vi "Load Becker-Hickl File Setup.vi"(8 "Error In":errorcluster, 9 "Setup Length":i16, 10 "Setup Offset":i32, 11 "File Path Control":path) -> (0 "Error Out":errorcluster, 1 "TAC Parameters":T3 {"Frequency (Hz)" format="%#.6g"; "TAC Range (s)" format="%.6g"; "TAC Bin (s)" format="%#.6g"}, 2 "Image Parameters":T2, 3 "File Path out":path, 4 "Image Sizes":T1)   [LabVIEW 2021, in "Becker-Hickl Files.lvlib"]
uses:
  Becker-Hickl Files.lvlib
  Becker-Hickl TAC Parameters.ctl
  Becker-Hickl Image Parameters.ctl
  Becker-Hickl FLIM Image Sizes.ctl
panel:
  out "Setup Binary Data String":string
  out "Setup Data String":string
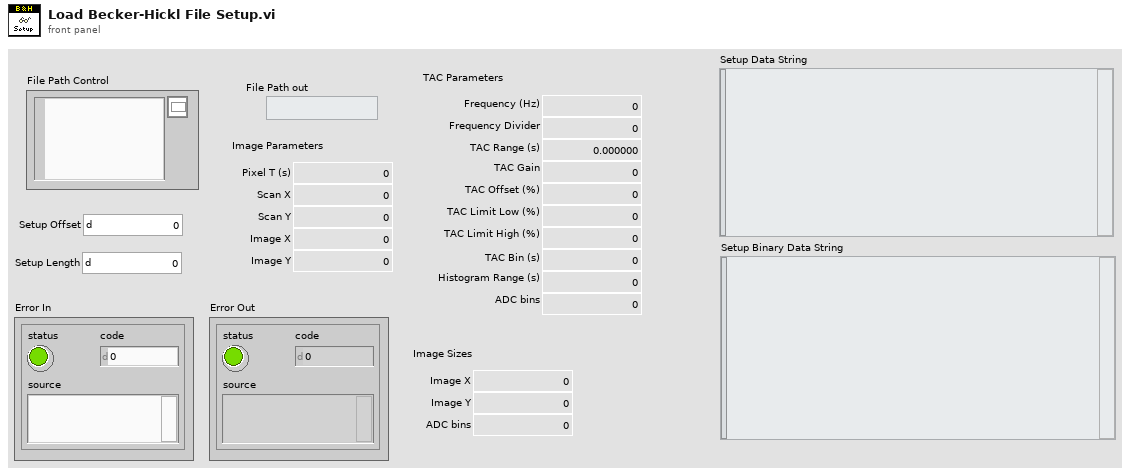
[diagram p1: front panel]
types:
  T1 = typedef "Becker-Hickl Files.lvlib/Becker-Hickl FLIM Image Sizes.ctl" = cluster{"Image X":i32, "Image Y":i32, "ADC bins":i32}
  T2 = typedef "Becker-Hickl Files.lvlib/Becker-Hickl Image Parameters.ctl" = cluster{"Pixel T (s)":dbl, "Scan X":i32, "Scan Y":i32, "Image X":i32, "Image Y":i32}
  T3 = typedef "Becker-Hickl Files.lvlib/Becker-Hickl TAC Parameters.ctl" = cluster{"Frequency (Hz)":dbl, "Frequency Divider":i32, "TAC Range (s)":dbl, "TAC Gain":i32, "TAC Offset (%)":dbl, "TAC Limit Low (%)":dbl, "TAC Limit High (%)":dbl, "TAC Bin (s)":dbl, "ADC bins":i32, "Histogram Range (s)":dbl}
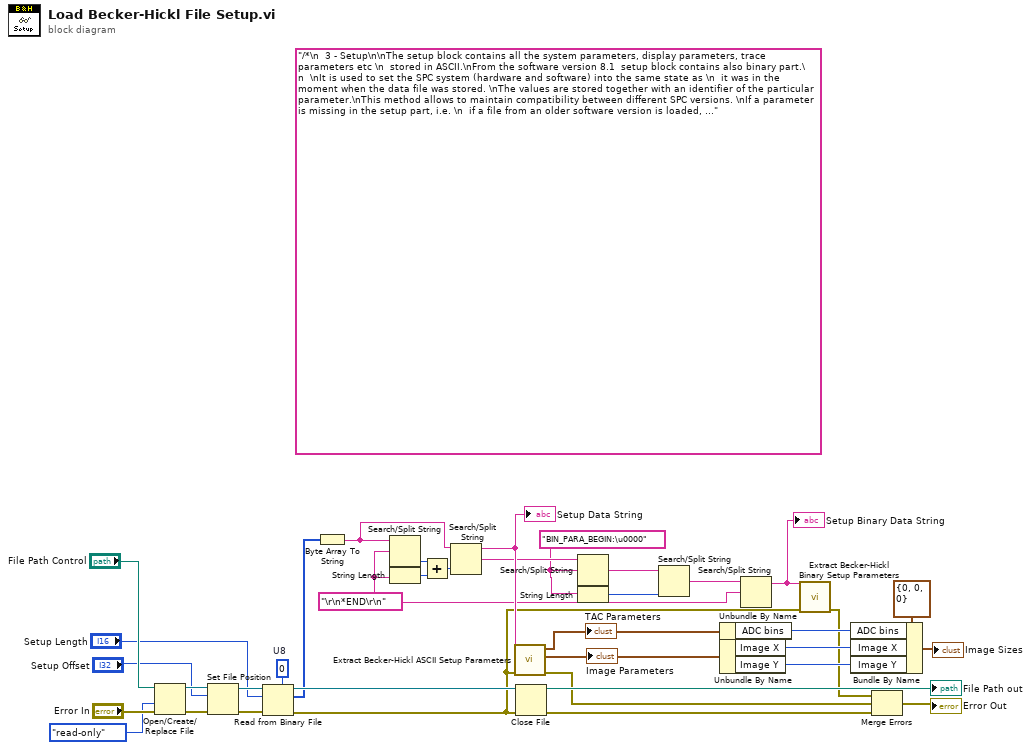
[diagram p0: block diagram]
diagram:
  w6 = "BIN_PARA_BEGIN:\u0000" ("search string/char (-)")
  w3 = "\r\n*END\r\n" ("search string/char (-)")
  w37 = u8 0  # U8
  (unwired) "/*\n  3 - Setup\n\nThe setup block contains all the system parameters, display parameters, trace parameters etc \n  stored in ASCII.\nFrom the software version 8.1  setup block contains also binary part.\n  \nIt is used to set the SPC system (hardware and software) into the same state as \n  it was in the moment when the data file was stored. \nThe values are stored together with an identifier of the particular parameter.\nThis method allows to maintain compatibility between different SPC versions. \nIf a parameter is missing in the setup part, i.e. \n  if a file from an older software version is loaded, a default value is used \n   when the file is loaded. \nFor Multi SPC Systems the system parameters section contains subsections \n   for module parameters which are separate for the individual modules.\n\nASCII part of the setup block starts with the line\n*SETUP\nand ends with the line\n*END\n\nAfter this  binary part of the setup follows  ( for the files created with the software\n  version 8.1 and next ) \n\nIt starts with the text BIN_PARA_BEGIN\nDirectly after BIN_PARA_BEGIN text comes:\n  -  4-byte value which is equal to the length of binary setup \n          ( all suqsequent headers and structures up to *END text )\n  -  BHBinHdr bh_bin_hdr       \n  -  SPCBinHdr spc_bin_hdr       \n  -  structures defined in spc_bin_hdr header\n\nbinary setup ends with the line\n*END\n\nbinary setup contains mainly display parameters for different graph windows\n ( Main graph (2D, 3D), FCS and other (in future) ), \n which are used by the main software to restore display parameters\n   of the specific windows\n DI_ parameters in ASCII part of the setup are now obsolete and are present\n for compatibility reason only\n*/\n\ntypedef struct {\n   unsigned long     soft_rev;       // software revision\n   unsigned long     para_length;    // currently set to 0 \n   unsigned long     reserved1;\n   unsigned short    reserved2;\n   }BHBinHdr;\n\n\n// all offsets are given from the beginning of the file\n// all parts lengths are given in bytes\n\ntypedef struct {\n  unsigned long  FCS_old_offs;    // offset of FCSParam structure for FCS parameters\n  unsigned long  FCS_old_size;    //  FCSParam structure size\n               //  FCSParam is obsolete - needed only for compatibility\n               //  with software v. 8.1 - 8.2\n               //  from v.8.3 FCS parameters are included further in HSTParam \n  unsigned long  gr1_offs;    // offset of GR_Param structure for main graph window\n  unsigned long  gr1_size;    //  GR_Param structure size                       \n  unsigned long  FCS_offs;    // offset of HSTParam structure for FCS parameters\n  unsigned long  FCS_size;    //  HSTParam structure size\n  unsigned long  FIDA_offs;   // offset of HSTParam structure for FIDA window parameters\n  unsigned long  FIDA_size;   //  HSTParam structure size \n  unsigned long  FILDA_offs;  // offset of HSTParam structure for FILDA window parameters\n  unsigned long  FILDA_size;  //  HSTParam structure size\n  unsigned long  gr2_offs;    // offset of GR_Param structure for the 1st additional graph\n  unsigned short gr_no;       // number of additional GR_Param structures, ( size = gr1_size )\n  unsigned short hst_no;      // number of additional HSTParam structures, ( size = FCS_size )\n  unsigned long  hst_offs;    // offset of the 1st additional HSTParam structure\n  unsigned long  GVD_offs;    // offset of GVDParam structure for GVD-120 parameters \n  unsigned short GVD_size;    //  GVDParam structure size\n  unsigned short FIT_offs;    // offset of FITSetup structure for FIT parameters\n  unsigned short FIT_size;    //  FITSetup structure size\n  unsigned short extdev_offs;  // offset of external devices setup structures\n  unsigned short extdev_size;  //  size of external devices setup structures\n  unsigned short reserve2;\n  unsigned long  reserve3;\n  }SPCBinHdr;\n\n/*\nSPCBinHdr header includes offsets of GR_Param structure for the main display window\n  and HSTParam structures for FCS, FIDA and FILDA windows.\nAnother GR_Param structures can be included if additional 3D display windows were \n  opened\nAnother HSTParam structures can be included if additional histograms windows were \n  opened ( e.g. MCS (Macro Time) histogram )\nGVDParam structure contains parameters of GVD-120 module which controls BH Galvano Scanner.\nFITParam structure contains start values of FCS fitting parameters   \nOther fields will be used in future software versions\nFCS, FIDA, FILDA, MCS windows parameters are defined below in HSTParam structure\nThe structure contains attributes of histogram display windows,\n  which can be visible in FIFO mode\n*/\n\ntypedef struct {\n  int   top;\n  int   left;\n  int   height;\n  int   width;\n  int   flags;  // 0x1 - visible\n  }BHPanelAttr;\n\n\n\ntypedef union \n{\n  int             i;\n  unsigned int    u;\n  int             b;\n  short           h;\n  unsigned short  g;\n  long            l;\n  unsigned long   m;\n  float           f;\n  double          d;\n  char            c;\n} DparVal;\n\n\n\n  \n  \ntypedef struct            \n{\n  DparVal maxcnt;     //  DI_MAXCNT    \n  DparVal lbline;     //  DI_LBLINE  \n  DparVal bline;      //  DI_BLINE     \n  int  scale;         //  DI_SCALE   \n  int  grid;          //  DI_GRID  X : bit1, bit3 minor/ Y : bit2, bit 4 minor/ bit0 = X+Y\n  int  plot_style;    //  DI_TRACE     \n  int  point_style;   //  DI_PSTYLE    \n  int  line_style;    //  set to 0    \n  int  point_freq;    //  DI_PFREQ   \n  int  resize;        //  0 - not set, 1- Full size, 2 - Proportional, 3- other\n  int   grid_color;   //  DI_GCOL_F\n  int   bkg_color;    //  DI_GCOL_B\n  int   d2_mode;      //  DI_2DDIS\n  short reverse;      //  DI_XREV - bit 0, DI_YREV - bit 1                          \n  short ascale;       //  autoscale for 2D\n  DparVal xlow;          \n  DparVal xhigh;          \n  int  xscale;        //  Xscale log = 1\n  DparVal yhilim;     // high limit for y scale  \n} Disp2DAttr;\n\n\n\n\ntypedef struct  {    // obsolete, needed only for compatibility with software v. 8.1 - 8.2\n  int      view_decay;      \n  int      view_fcs;   \n  float    cortime; // correlation time [ms] \n  BHPanelAttr  pnl_attr; \n  Disp2DAttr   d2para;\n  }FCSParam;\n\n\n// Histogram traces parameters ( FCS, FIDA, FILDA, MCS )\ntypedef struct  {\n  short    active;         // (0)1 - (not) active   \n  short    module;\n  short    curve;          // routing channel no \n  short    cross_curve;    // cross correlation channel number for FCS\n                      //    ( when = curve and module = cross_module -  auto FCS )\n  short    cross_module;   // cross correlation module number for FCS\n  int      color;          // trace color\n  int      points;         // number of points in trace \n  }HSTtrace;  //\n\n\n\n#define MAX_NO_OF_TRACES  8\n\ntypedef struct{        // structure for FCS, FIDA and FILDA histogram windows\n  int              active;   // window visible, histogram is calculated\n  unsigned short   hst_type; // additional histogram parameters\n                    // for FCS:  0 - linear FCS with log binning ( 100 bins/log )\n                              // when bit 15 = 1 ( 0x8000 ) - Multi-Tau FCS \n                              //           where bits 14-0 = ktau parameter\n  short          reserve;   \n  float          time;     // in [ms], correlation time for FCS, \n                           // period time for FIDA, FILDA, time per point for MT\n  BHPanelAttr    pnl_attr; \n  Disp2DAttr     d2para;\n  HSTtrace       htrace[MAX_NO_OF_TRACES];\n  }HSTParam;\n\n\n\n#define MAX_NO_OF_COLORS   11 // max value for DI_COL_NO\n\ntypedef struct            \n{\n  int   offsx;             //  DI_3DOFFX - offset X for 3D display \n  int   offsy;             //  DI_3DOFFY - offset Y for 3D display         \n  int   inclination;       //  DI_3DINCX - inclination X for 3D display    \n  int   body_color;        //  DI_BOD_C\n  int   curve_color;       //  DI_3DCOL\n  int   d3_mode;           //  DI_3DMODE\n  int   ywin;              //  DI_YWIN  \n  int   xwin;              //  DI_XWIN  \n  int   twin;              //  DI_TWIN  \n  int   sywin;             //  DI_SYWIN  \n  int   sxwin;             //  DI_SXWIN  \n  int   d3_style;          //  DI_3DSTYL\n  int   interpolate;       //  DI_INTCOL- bit 0, DI_INTPIX - bit 1\n  int   col_no;            //  DI_COL_NO\n  int   color[MAX_NO_OF_COLORS];   // 0 - DI_COLMIN, 1 - DI_COLMAX, 2..5 - DI_COL2-5,\n                           // 6 - 10 are stored in BIN_SETUP\n  int   col_hi;            //  DI_HICOL\n  int   detail;            //  DI_DETAIL  \n  int   ascale;            //  DI_ASCALE  \n  int   lcol_no;           //  DI_COL_NO  for log scale\n} Disp3DAttr;\n\n\n\ntypedef struct _Interval {\n    unsigned int    from;\n    unsigned int    to;\n    }Interval;\n\n\n\ntypedef struct _Trace3d {\n  short    log_scale;       /*  display type 0- linear , 1- logarithmic  */\n  short    offsx;           /*  display offset X  - parameter DI_3DOFFX  */\n  short    offsy;           /*  display offset Y  - parameter DI_3DOFFY  */\n  double   inclination;     /*  display inclination- parameter DI_3DINCX  */\n  short    mode;            /*  display mode  - parameter DI_3DMODE  */\n  unsigned int    page;            /*  page number in SPC memory */\n  unsigned int    no_of_curves;    /*  number of curves  */\n  unsigned int    no_of_disp_curves;    /*  number of displayed curves */\n  unsigned int    no_of_points;    /*  number of points  */\n  short    resolution; \n  Interval * win;            /*  pointer to  window interval - depending on\n                                   display mode = DI_XWIN,DI_YWIN,DI_TWIN */\n  Interval * win_y;          /*  pointer to Y window interval - for f(t,x,y,param) */\n  unsigned short  first_disp_point; /*  number of first displayed point on curves  */\n  unsigned short  last_disp_point;  /*  number of last displayed point on curves  */\n  unsigned int    first_disp_curve; /*  number of first displayed curve  */\n  unsigned int    last_disp_curve;  /*  number of last displayed curve  */\n  short    reduction;        /*  display reduction ratio  */\n  int      color;            /*  colors of curves  (DIS_3DCOL converted ) */\n  int      body_color;       /*  color of the body (DIS_BOD_C converted ) */\n  double   curve1_xpos;      /*  x position on the graph of the first curve */\n  double   curve1_ypos;      /*  y position on the graph of the first curve */\n  double   xinc;             /*  x increment */\n  double   yinc;             /*  y increment */\n  double   ygain;            /*  y gain */\n  short    no;               /*  3d trace no */\n  short    sreserve;         /*  for future use */\n  unsigned long    reserve;  /*  for future use */\n  long     low_offset;       /*  DI_BLINE */\n  long     max_count;        /*  DI_MAXCNT */\n  Interval * swin;           /*  pointer to ScanX(Y) window interval -  depending on\n                                 display mode = DI_XWIN,DI_YWIN,DI_TWIN */\n  Interval * swin_y;         /*  pointer to ScanY window interval  */\n  long no_of_blocks;         /*  for get3Dcurve */\n  } Trace3d;\n\n\n\ntypedef struct  {\n  short               active;      \n  unsigned short      tr3d_module; // mod_no for 3D trace, missing in Trace3d structure\n  unsigned short      mem_bank;      \n  unsigned short      reserved2;      \n  double              dreserved1;\n  double              dreserved2;\n  BHPanelAttr         pnl_attr; \n  Disp2DAttr          d2para;    // Disp2DAttr for modes with 2D display  \n  Disp3DAttr          d3para;    // additional parameters for 3D display  \n  Disp2DAttr          d23para;   // Disp2DAttr for modes with 3D display  \n  Trace3d             tr3d;      // 3D trace parameters structure                                      \n  Disp2DAttr          d21para;   // Disp2DAttr for modes with 2D display and 32-bit range\n                                 //      ( fifo modes & 2D Block Display )\n  }GR_Param;                     // Main Graph window parameters\n\n"
  n1 = Open/Create/Replace File(file path (use dialog)="File Path Control", error in="Error In", access (0:read/write)=enum16{"read/write", "read-only", "write-only"}."read-only") -> (refnum out=w35:refnum<file>, error out=w36:errorcluster)  [unwired: 3 in, 1 out]
  n2 = Set File Position(offset (in bytes) (0)="Setup Offset", refnum=w35, error in=w36) -> (refnum out=w34:refnum<file>, error out=w33:errorcluster)  [unwired: 1 in]
  n3 = Read from Binary File(5:w37, 8:w33, 10:"Setup Length", 11:w34) -> (0:w10:errorcluster, 2:w26:u8[], 3:w32:refnum<file>)  [unwired: 2 in, 1 out]
  n4 = Byte Array To String(unsigned byte array=w26) -> (string=w20:string)
  n5 = Search/Split String(string=w20, search string/char (-)=w3) -> (offset of match=w23:i32)  [unwired: 1 in, 2 out]
  n6 = String Length(string=w3) -> (length=w22:i32)
  n7 = Add(x=w23, y=w22) -> (x+y=w21:i32)
  n8 = Search/Split String(string=w20, offset (0)=w21) -> (substring before match=w19:string, match + rest of string=w11:string)  [unwired: 1 in, 1 out]
  "Setup Data String" <- w19
  n9 = call "Extract Becker-Hickl ASCII Setup Parameters.vi"("Error In"=w10, "B&H Setup String"=w19) -> ("Error Out"=w7:errorcluster, "Image Parameters"=w17:T2, "TAC Parameters"=w18:T3)  [unwired: 7 in]
  "TAC Parameters" <- w18
  "Image Parameters" <- w17
  n10 = Close File(refnum=w32, error in=w10) -> (path=→"File Path out":path, error out=w24:errorcluster)
  n11 = Search/Split String(string=w11, search string/char (-)=w6) -> (match + rest of string=w5:string)  [unwired: 1 in, 2 out]
  n12 = String Length(string=w6) -> (length=w1:i32)
  n13 = Search/Split String(string=w5, offset (0)=w1) -> (match + rest of string=w4:string)  [unwired: 1 in, 2 out]
  n14 = Unbundle By Name(w18) -> ("ADC bins"=w15:i32)
  n15 = Unbundle By Name(w17) -> ("Image X"=w14:i32, "Image Y"=w13:i32)
  n16 = Search/Split String(string=w4, search string/char (-)=w3) -> (substring before match=w2:string)  [unwired: 1 in, 2 out]
  "Setup Binary Data String" <- w2
  n17 = call "Extract Becker-Hickl Binary Setup Parameters.vi"("Error In"=w10, "B&H Setup String"=w2) -> ("Error Out"=w8:errorcluster)  [unwired: 9 in]
  n18 = Bundle By Name(cluster=T1 {"Image X"=0, "Image Y"=0, "ADC bins"=0} ("Image Sizes"), "ADC bins"=w15, "Image X"=w14, "Image Y"=w13) -> (→"Image Sizes":T1)
  n19 = Merge Errors(w8, w7, w24) -> (→"Error Out":errorcluster)
